vi "oax_Extract Channel Property and Convert to DAQ Config Cluster.vi"(8 "error in (no error)":errorcluster, 10 "rotating direction":u16(ring) items=["CCW", "CW"], 11 "MCM DAQ Config":T4 {"probe angle [deg]" max=360; "pregain" format="%.2f"; "IEPE" items=["On", "Off", "None"]; "coupling" items=["DC", "AC"]; "engineering units" items=["custom..."=0, "V"=1, "A"=21, "C"=30, "pC"=31, "s"=32, "-"=29, "Pa"=2, "N"=20, "g"=3, "m/s^2"=4, "m/s"=5, "m"=6, "mm/s"=12, "mm"=13, "micron/s"=14, "micron"=15, "in/s^2"=7, "in/s"=8, "in"=9, "mil/s"=10, "mil"=11, "rad/s^2"=16, "rad/s"=17, "rad"=18, "deg/s^2"=26, "deg/s"=27, "deg"=28, "RPM"=22, "cycle/s^2"=23, "Hz"=24, "cycle"=25, "strain"=19]; "sensor sensitivity (mV/EU)" format="%.2f"; "dB reference" format="%.1e"}) -> (0 "error out":errorcluster, 2 "channel properties":T1[](array[typedef]) {"probe angle [deg]" max=360; "direction" items=["CCW", "CW"]}, 3 "DAQ Config":T2 {"pregain" format="%.2f"; "IEPE" items=["On", "Off", "None"]; "coupling" items=["DC", "AC"]; "engineering units" items=["custom..."=0, "V"=1, "A"=21, "C"=30, "pC"=31, "s"=32, "-"=29, "Pa"=2, "N"=20, "g"=3, "m/s^2"=4, "m/s"=5, "m"=6, "mm/s"=12, "mm"=13, "micron/s"=14, "micron"=15, "in/s^2"=7, "in/s"=8, "in"=9, "mil/s"=10, "mil"=11, "rad/s^2"=16, "rad/s"=17, "rad"=18, "deg/s^2"=26, "deg/s"=27, "deg"=28, "RPM"=22, "cycle/s^2"=23, "Hz"=24, "cycle"=25, "strain"=19]; "sensor sensitivity (mV/EU)" format="%.2f"; "dB reference" format="%.1e"})   [LabVIEW 2017]
uses:
  <vilib>/addons/Sound and Vibration/Order Analysis/Example Support/sub VIs/OAXML_DSA MCM DAQ Config.ctl
  <vilib>/addons/_NISVFA/_Shared subVIs/Controls/svc_Engineering Units Text Ring.ctl
  <vilib>/addons/Sound and Vibration/Order Analysis/Example Support/sub VIs/OAXML_DSA DAQ Config.ctl
  <vilib>/addons/Sound and Vibration/Order Analysis/Data Presentation/SubVIs/OAT MCM Channel Property.ctl
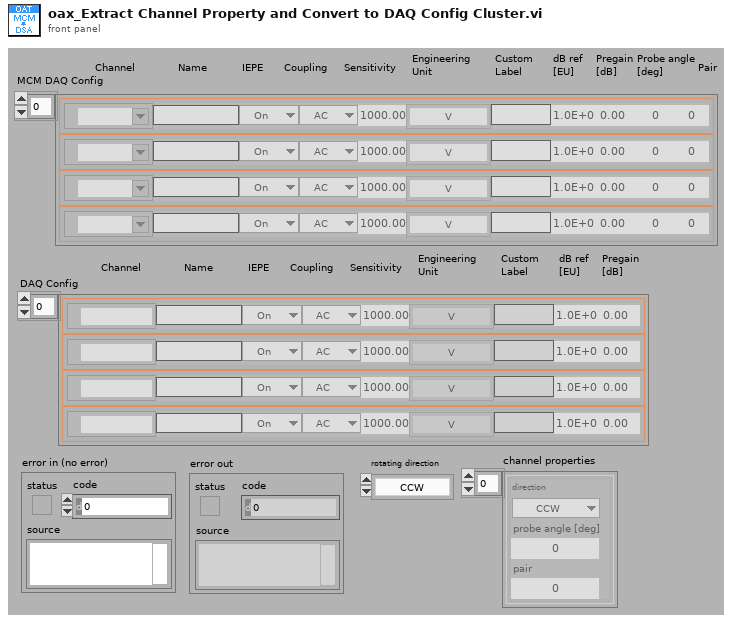
[diagram p1: front panel]
types:
  T1 = typedef "OAT MCM Channel Property.ctl" = cluster{"direction":u16, "probe angle [deg]":u16, "pair":u16}
  T2 = typedef "OAXML_DSA DAQ Config.ctl" = cluster{"name":string, "channel":tag, "coupling":u16, "dB reference":sgl, "sensor sensitivity (mV/EU)":dbl, "engineering units":T3, "IEPE":u16, "custom label":string, "pregain":sgl}[]
  T3 = typedef "svc_Engineering Units Text Ring.ctl" = u16
  T4 = typedef "OAXML_DSA MCM DAQ Config.ctl" = cluster{"name":string, "channel":tag, "coupling":u16, "dB reference":sgl, "sensor sensitivity (mV/EU)":dbl, "engineering units":T3, "IEPE":u16, "custom label":string, "pregain":sgl, "probe angle [deg]":u16, "pair":u16}[]
  T5 = cluster{"name":string, "channel":tag, "coupling":u16, "dB reference":sgl, "sensor sensitivity (mV/EU)":dbl, "engineering units":T3, "IEPE":u16, "custom label":string, "pregain":sgl}
  T6 = cluster{"rotating direction":u16, "probe angle [deg]":u16, "pair":u16}
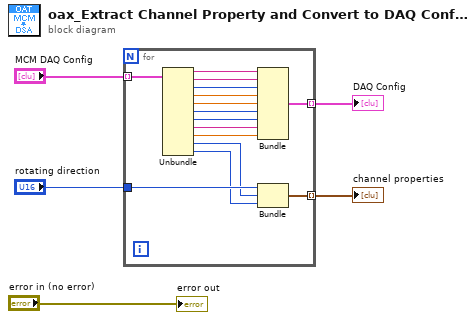
[diagram p0: block diagram]
diagram:
  n1 = for {
    tunnel: "MCM DAQ Config" -> [w20] mode=indexing
    tunnel: "rotating direction" -> [w10]
    tunnel: [w7] -> w3 mode=indexing
    tunnel: [w6] -> w2 mode=indexing
    n2 = Unbundle(w20) -> ("name"=w19:string, "channel"=w18:tag, "coupling"=w17:u16, "dB reference"=w16:sgl, "sensor sensitivity (mV/EU)"=w15:dbl, "engineering units"=w14:T3, "IEPE"=w13:u16, "custom label"=w12:string, "pregain"=w11:sgl, "probe angle [deg]"=w9:u16, "pair"=w8:u16)
    n3 = Bundle("name"=w19, "channel"=w18, "coupling"=w17, "dB reference"=w16, "sensor sensitivity (mV/EU)"=w15, "engineering units"=w14, "IEPE"=w13, "custom label"=w12, "pregain"=w11) -> (w7:T5)  [unwired: 1 in]
    n4 = Bundle("rotating direction"=w10, "probe angle [deg]"=w9, "pair"=w8) -> (w6:T6)  [unwired: 1 in]
  }
  "DAQ Config" <- w3
  "channel properties" <- w2
  "error out" <- "error in (no error)"
